vi "创建RAG知识库.vi"(11 "init base£":bool=TRUE) -> ()   [LabVIEW 2023, in "LabVIEW RAG.lvlib"]
uses:
  RAG_LV_API/LabVIEW RAG.lvlib
  RAG_LV_API/Typedefs/RAG Chunk Settings.ctl
  labview-ai-share/LabVIEW AI Base.lvlib
panel:
  in  "Tab Control":enum32{"Standard Settings", "Advanced Settings"}(tab)
  in  "PDF Folder to Build KB":path
  in  "Markdown Folder to Build KB":path
  in  "Knowledge Base Name":string="NI-cDAQ"
  in  "Embedding Model Base URL":string(combo)="http://10.144.128.8:1234/v1"
  in  "Embedding Model":string(combo)="mixedbread-ai/mxbai-embed-large-v1"
  in  "Clear DB?":bool=TRUE
  out "error out":errorcluster
  in  "Chunk Settings":T1={"Chunk Size"=1000, "Chunk Overlap"=100}
  in  "Generate":bool
  in  "STOP":bool
  in  "Python venv path":path=path "C:/dev/labview-ai"
  in  "Chroma Database Folder":path=path "C:/chroma_db"
  in  "Python version":string="3.10"
  # "创建RAG知识库"
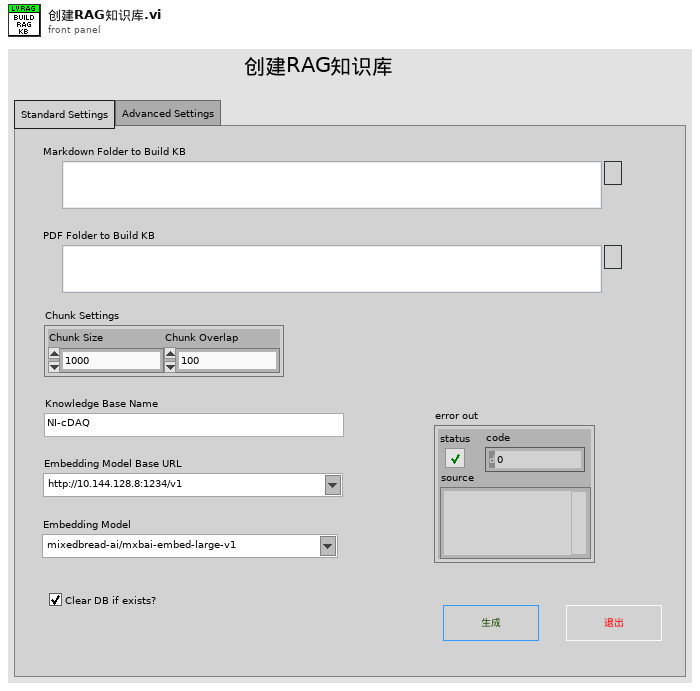
[diagram p1: front panel]
types:
  T1 = typedef "LabVIEW RAG.lvlib/RAG Chunk Settings.ctl" = cluster{"Chunk Size":u32, "Chunk Overlap":u32}
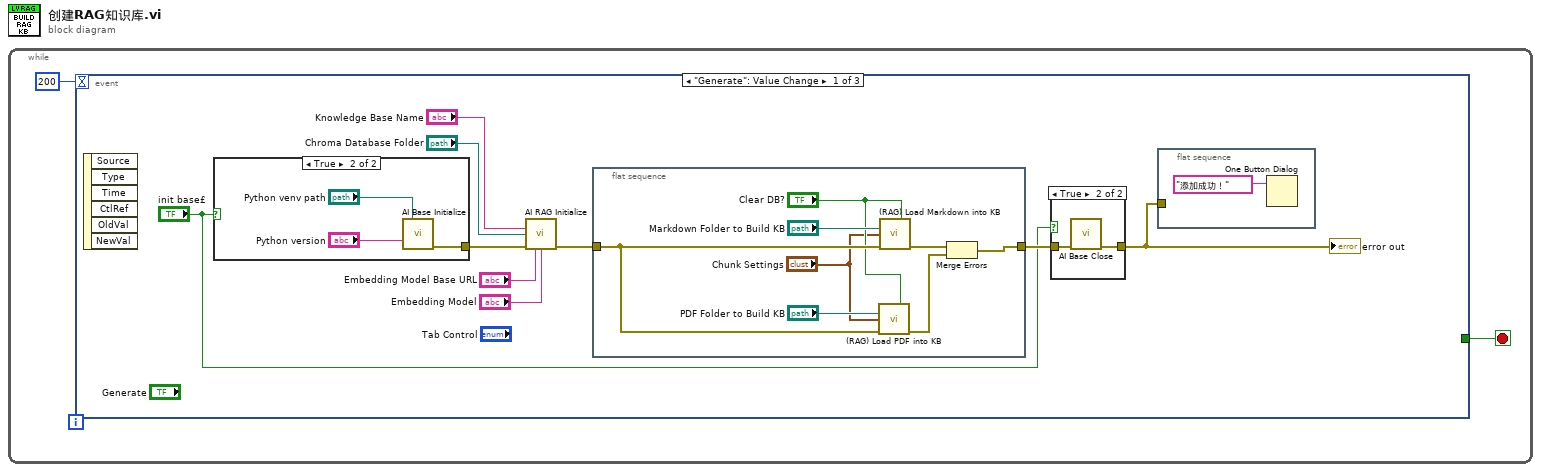
[diagram p0: block diagram]
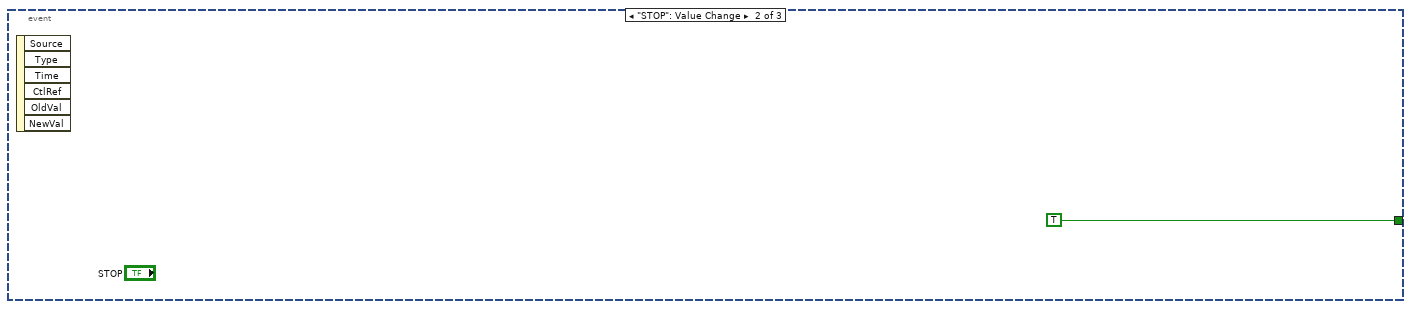
[diagram p4: hidden frame]
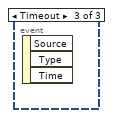
[diagram p5: hidden frame]
diagram:
  n1 = while {
    stop <- w1 stop-if-true
    n2 = event shown="[0] \"Generate\": Value Change" {
      selector: _ -> [_ _ _]
      dyn-events: _ -> [_ _ _]
      timeout: 200 -> [_ _ _]
      tunnel: [_ TRUE _] -> w1
      event "Generate": Value Change {
        n3 = event-data() -> ()  [unwired: 1 in, 6 out]
        n4 = case shown="True" "init base£" {
          tunnel: [_ w26] -> w11
          frame False {
          }
          frame True {
            n5 = call "AI Base Initialize.vi"("Python venv path"="Python venv path", "Python version"="Python version") -> ("error out"=w26:errorcluster)  [unwired: 11 in, 2 out]
          }
        }
        n6 = call "AI RAG Initialize.vi"("Knowledge Base Name"="Knowledge Base Name", "Chroma Database Folder"="Chroma Database Folder", "error in (no error)"=w11, "Embedding Model URL"="Embedding Model Base URL", "Embedding Model Name"="Embedding Model") -> ("error out"=w9:errorcluster)  [unwired: 10 in]
        n7 = flat-sequence {
          tunnel: [w15] -> w10
          tunnel: w9 -> [w18]
          frame #0 {
            n8 = call "(RAG) Load PDF into KB.vi"("Clear DB?"="Clear DB?", "PDF Folder to Build KB"="PDF Folder to Build KB", "Chunk Settings"="Chunk Settings", "error in"=w18) -> ("error out"=w14:errorcluster)  [unwired: 9 in, 2 out]
            n9 = call "(RAG) Load Markdown into KB.vi"("Clear DB?"="Clear DB?", "Markdown Folder to Build KB"="Markdown Folder to Build KB", "Chunk Settings"="Chunk Settings", "error in"=w18) -> ("error out"=w20:errorcluster)  [unwired: 10 in, 1 out]
            n10 = Merge Errors(w20, w14) -> (w15:errorcluster)
          }
        }
        n11 = case shown="True" "init base£" {
          tunnel: w10 -> [w21 w23]
          tunnel: [w21 w22] -> w3
          frame False {
          }
          frame True {
            n12 = call "AI Base Close.vi"("error in"=w23) -> ("error out"=w22:errorcluster)  [unwired: 10 in]
          }
        }
        "error out" <- w3
        n13 = flat-sequence {
          tunnel: w3 -> [_]
          frame #0 {
            n14 = One Button Dialog(message="添加成功！") -> ()  [unwired: 1 in, 1 out]
          }
        }
      }
      event "STOP": Value Change {
        n15 = event-data() -> ()  [unwired: 1 in, 6 out]
      }
      event Timeout {
        n16 = event-data() -> ()  [unwired: 1 in, 3 out]
      }
    }
  }
